vi "Evaluate Part 1.vi"() -> ()   [LabVIEW 2020]
uses:
  Memory Global.vi
  Numeric Keypad/Numeric Keypad.lvclass
panel:
  out "Answer":u64
  in  "Input":string
  # "337744744231414"
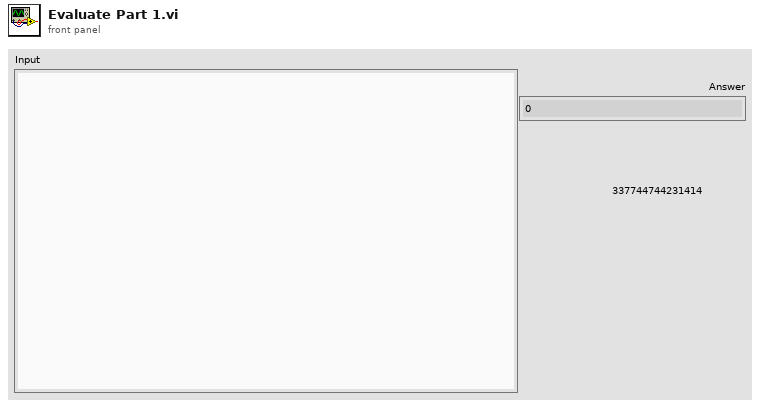
[diagram p1: front panel]
types:
  T1 = map{cluster{"Input":string, "Depth":u32, "Current position":string}, cluster{"default value":u64, "default value":string}}
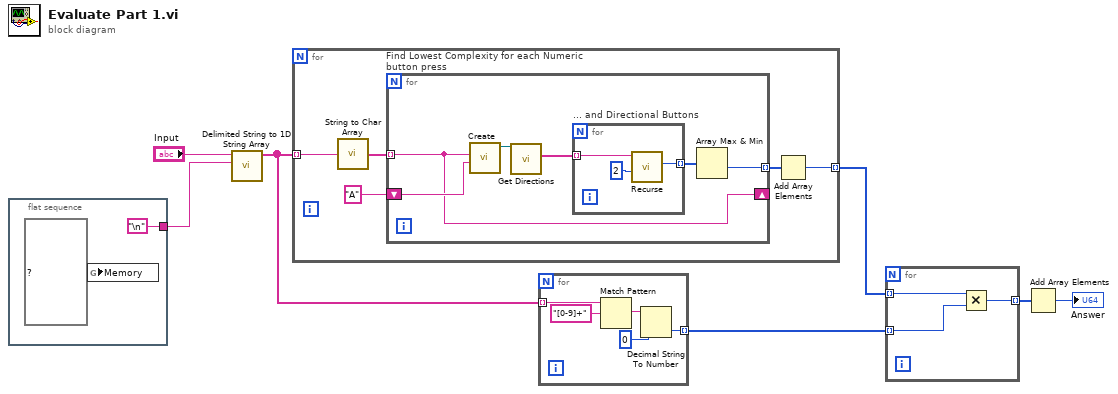
[diagram p0: block diagram]
diagram:
  n1 = flat-sequence {
    tunnel: ["\n"] -> w1
    frame #0 {
      n2 = global write "Memory Global.vi" "Memory"(T1 {} ("map")) -> ()
    }
  }
  n3 = call <vilib>:"Delimited String to 1D String Array.vi"("delimiter"=w1, "delimited string"="Input") -> ("string array"=w6:string[])  [unwired: 9 in]
  n4 = for {
    tunnel: w6 -> [w14] mode=indexing
    tunnel: [w11] -> w2 mode=indexing
    n5 = call "String to Char Array.vi"("Input"=w14) -> ("Array"=w12:string[])
    n6 = for "Find Lowest Complexity for each Numeric button press" {
      tunnel: [w17] -> w13 mode=indexing
      tunnel: w12 -> [w15] mode=indexing
      shift-right: [w15] -> _
      shift-left: "A" ("Current") -> [w16]
      n7 = call "Create.vi"("Current"=w16, "Input"=w15) -> ("Proto"=w20:refnum<class "Numeric Keypad.lvclass">)  [unwired: 9 in]
      n8 = call "Get Directions.vi"("Proto in"=w20) -> ("Directional Button Presses"=w19:string[])  [unwired: 9 in, 1 out]
      n9 = for "... and Directional Buttons" {
        tunnel: w19 -> [w23] mode=indexing
        tunnel: [w22] -> w18 mode=indexing
        n10 = call "Recurse.vi"("Depth"=u32 2, "Input"=w23) -> ("Complexity"=w22:u64)  [unwired: 8 in, 1 out]
      }
      n11 = Array Max & Min(array=w18) -> (min value=w17:u64)  [unwired: 3 out]
    }
    n12 = Add Array Elements(numeric array=w13) -> (sum=w11:u64)
  }
  n13 = for {
    tunnel: w6 -> [w28] mode=indexing
    tunnel: [w25] -> w5 mode=indexing
    n14 = Match Pattern(string=w28, regular expression="[0-9]+") -> (match substring=w26:string)  [unwired: 1 in, 3 out]
    n15 = Decimal String To Number(string=w26, default (0L)=u64 0 ("default (0 I32)")) -> (number=w25:u64)  [unwired: 1 in, 1 out]
  }
  n16 = for {
    tunnel: w5 -> [w31] mode=indexing
    tunnel: [w30] -> w4 mode=indexing
    tunnel: w2 -> [w29] mode=indexing
    n17 = Multiply(x=w29, y=w31) -> (x*y=w30:u64)
  }
  n18 = Add Array Elements(numeric array=w4) -> (sum=→"Answer":u64)
